vi "T1 new.vi"() -> ()   [LabVIEW 2012]
uses:
  <vilib>/DAQmx/read.llb/DAQmx Read (Counter U32 1Chan 1Samp).vi
  <vilib>/Analysis/1siggen.llb/Ramp Pattern by Samples.vi
  <vilib>/Utility/file.llb/Write To Spreadsheet File (DBL).vi
  <vilib>/Utility/file.llb/Write To Spreadsheet File (I64).vi
  <vilib>/DAQmx/create/channels.llb/DAQmx Create Channel (CI-Count Edges).vi
  <vilib>/DAQmx/configure/timing.llb/DAQmx Timing (Sample Clock).vi
  <vilib>/DAQmx/create/channels.llb/DAQmx Create Channel (CO-Pulse Generation-Ticks).vi
  <vilib>/DAQmx/configure/timing.llb/DAQmx Timing (Implicit).vi
  <vilib>/DAQmx/miscellaneous.llb/DAQmx Fill In Error Info.vi
  <resource>/objmgr/daqmx.rc
  <vilib>/Analysis/NI_AALBase.lvlib
panel:
  in  "N Cycles":i32
  in  "Sig/Ref Pause":dbl
  in  "file path (dialog if empty)":path
  in  "Z":dbl=0.001
  in  "Y":dbl=0.001
  in  "X":dbl=0.001
  out "Z Position":dbl=77.35
  out "Y Position":dbl=8.403706365395546
  out "X Position":dbl=39.29989668925261
  out "Cross Section Y":dbl[](graph)=[21.0, 21.0, 22.0, 23.0, 28.0, 18.0, 27.0, 23.0, 21.0, 23.0, 27.0, 24.0, 27.0, 48.0, 72.0, 155.0, 223.0, 269.0, 346.0, 310.0, 298.0, 201.0, 115.0, 77.0, 45.0, 31.0, 30.0, 22.0, 20.0, 22.0, 23.0, 32.0, 17.0, 24.0, 22.0, 22.0, 31.0, 30.0, 37.0]
  out "Cross Section X":dbl[](graph)=[40.0, 23.0, 29.0, 30.0, 20.0, 26.0, 17.0, 31.0, 49.0, 64.0, 98.0, 144.0, 182.0, 231.0, 269.0, 259.0, 260.0, 248.0, 193.0, 187.0, 133.0, 113.0, 84.0, 52.0, 39.0, 24.0, 24.0, 33.0, 19.0, 20.0, 16.0, 21.0, 26.0, 30.0, 25.0, 26.0, 20.0, 24.0, 24.0]
  out "Gave up?":bool
  in  "RS232 settings":cluster{"Portnumber":i32, "Baudrate":u16}={"Portnumber"=6, "Baudrate"=5} {"Portnumber" items=["COM1", "COM2", "COM3", "COM4", "COM5", "COM6", "COM7", "COM8", "COM9", "COM10", "COM11", "COM12", "COM13", "COM14", "COM15", "COM16", "COM17", "COM18", "COM19", "COM20", "COM21", "COM22", "COM23", "COM24", "COM25", "COM26", "COM27", "COM28", "COM29", "COM30"]; "Baudrate" items=["9600", "14400", "19200", "38400", "57600", "115200"]}
  in  "Y Parameters":T1={"Number of Y Steps"=200, "Max Y (V)"=2.0, "Min Y (V)"=-2.0}
  in  "X Parameters":T2={"Number of X Steps"=200, "Max X (V)"=2.0, "Min X (V)"=-2.0}
  in  "Path to spinapi.dll":path=path "C:/SpinCore/SpinAPI/dll/spinapi64.dll"
  in  "Pi Pulse?":bool
  in  "T1 AOM Rest":dbl=1e-06
  in  "Light Ratio":dbl=2.5e-06
  in  "T1 APD width":dbl=5e-07
  in  "T1 Signal Delay":dbl=6e-07
  in  "type 2":u16(ring)=1 items=["Linear", "Logarithmic"]
  in  "Tau No. Steps":i32=20
  in  "Tau Min":dbl=2e-08
  in  "Tau Max":dbl=0.001
  in  "Rabi Freq":dbl=7000000.0
  out "signal":u32
  out "ref":u32
  in  "samples per channel":i32=1000
  in  "N loops":i32=-1
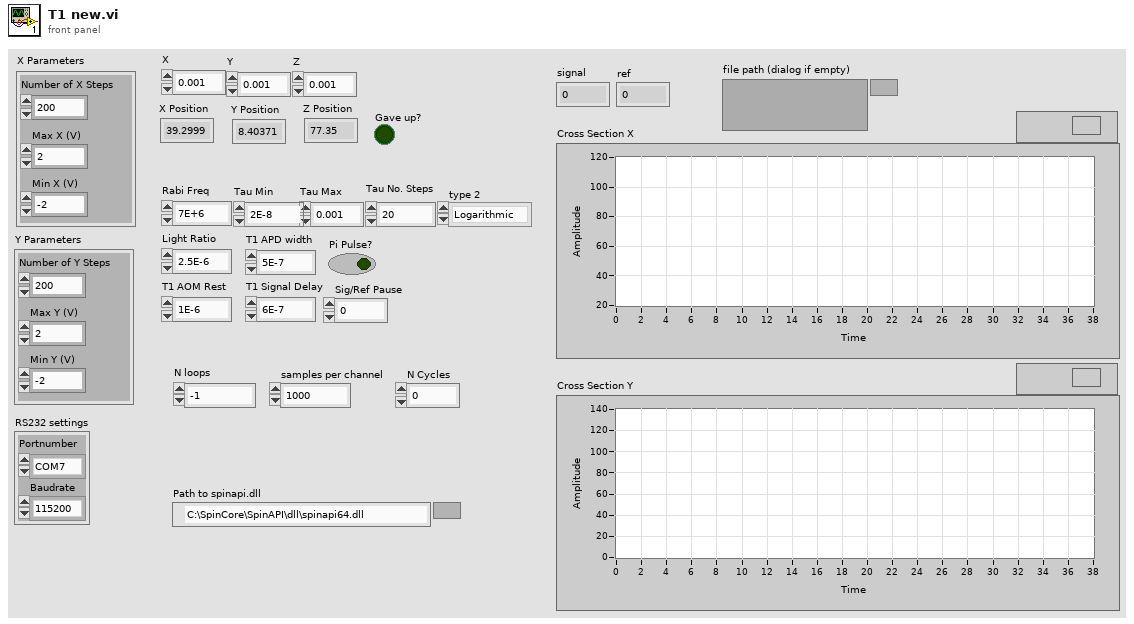
[diagram p1: front panel]
types:
  T1 = cluster{"Number of Y Steps":i32, "Max Y (V)":dbl, "Min Y (V)":dbl}
  T2 = cluster{"Number of X Steps":i32, "Max X (V)":dbl, "Min X (V)":dbl}
  T3 = enum16{"Pulse Program", "Frequency Registers", "TX Phase Registers", "RX Phase Registers"}
  T4 = cluster{"Instruct Data":i32, "Op Code":i32, "Flags":bool[], "Comments":string, "Time (s)":dbl}[]
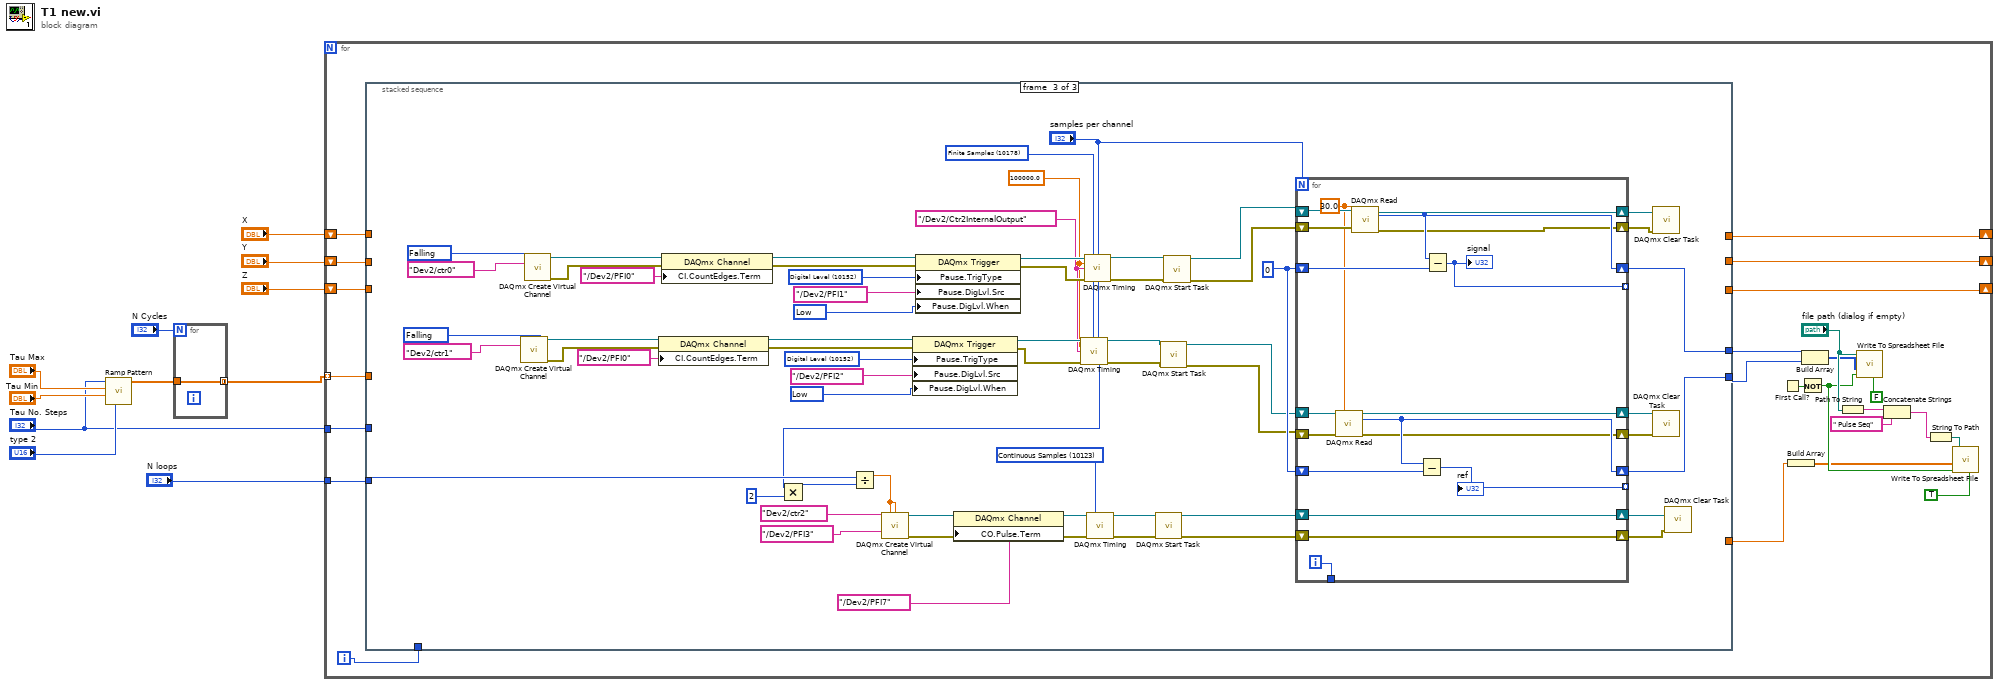
[diagram p0: block diagram]
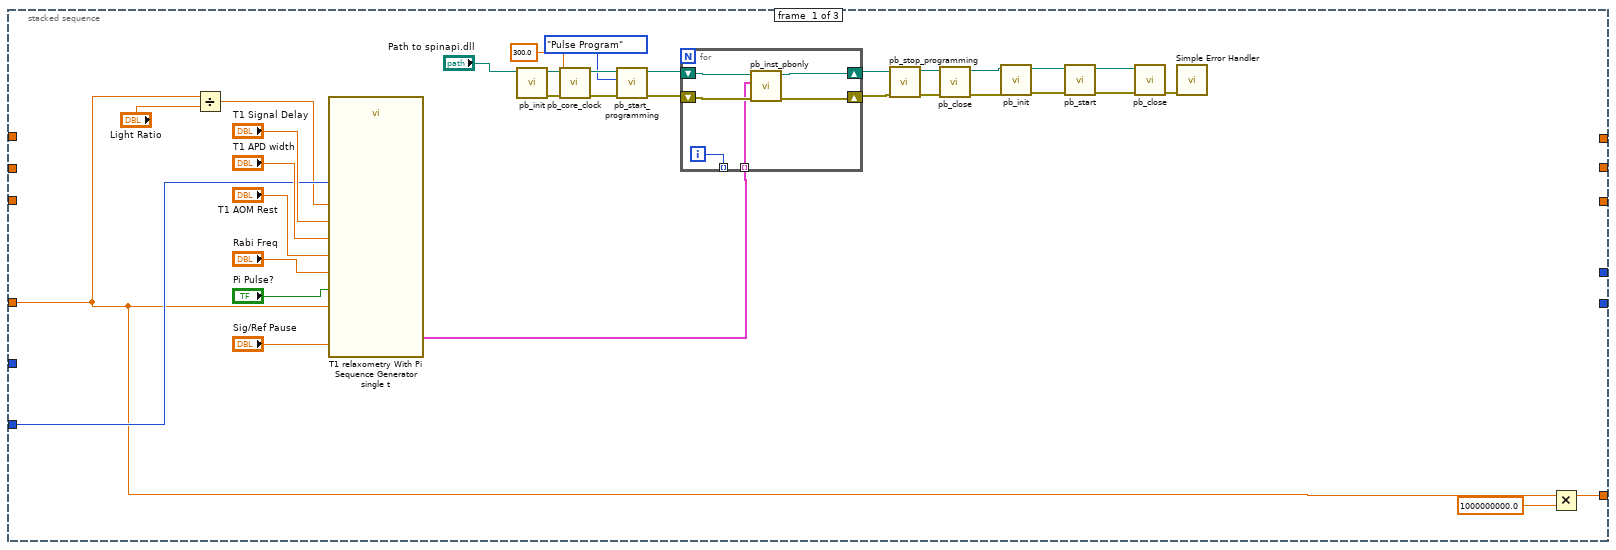
[diagram p2: hidden frame]
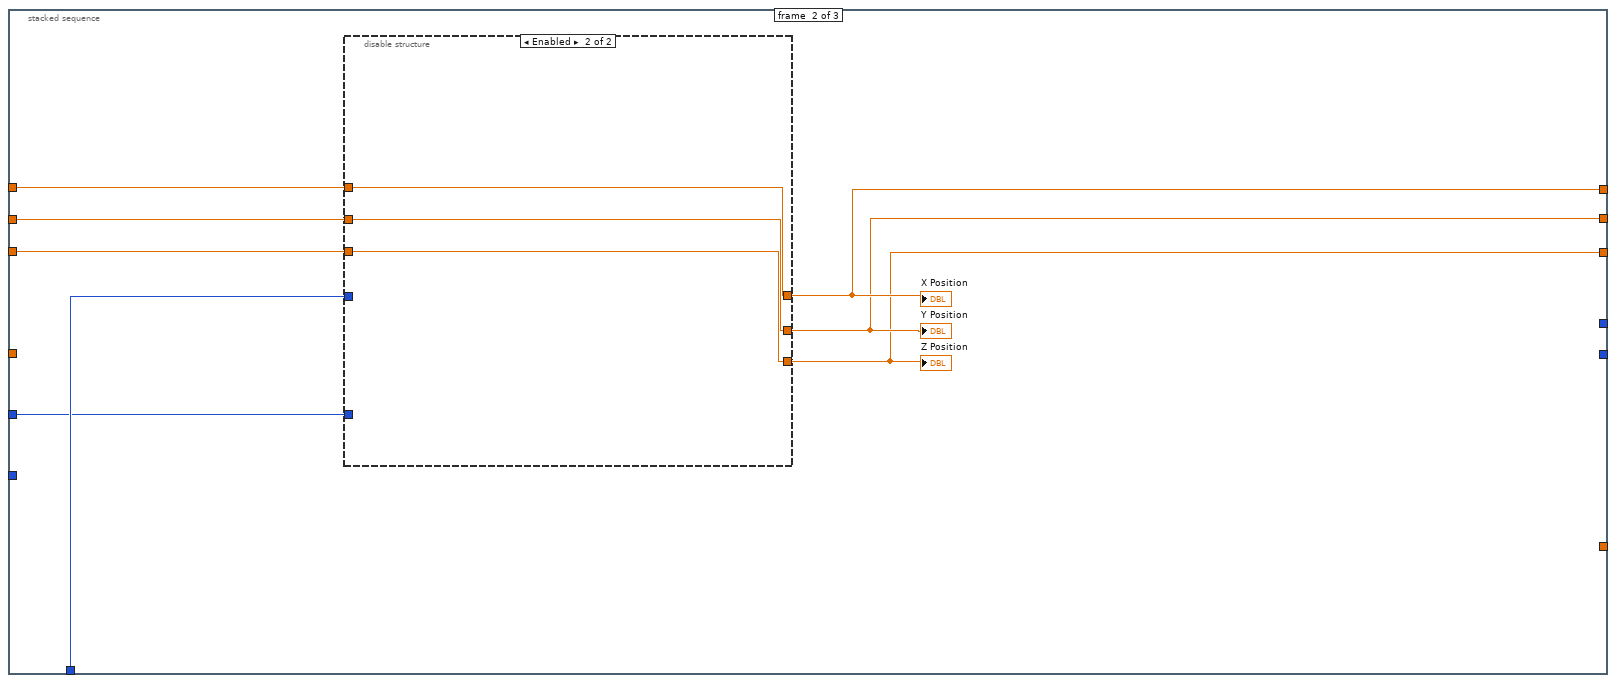
[diagram p3: hidden frame]
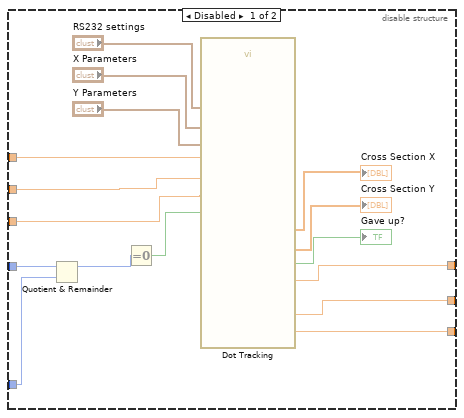
[diagram p4: hidden frame]
diagram:
  n1 = call-poly <vilib>:"Ramp Pattern.vi"("type"="type 2", "start"="Tau Min", "end"="Tau Max", "samples"="Tau No. Steps") -> ("Ramp Pattern"=w4:dbl[])  [unwired: 6 in, 1 out]
  n2 = for {
    N: "N Cycles" -> [_]
    tunnel: w4 -> [w12]
    tunnel: [w12] -> w3 mode=concatenating
  }
  n3 = for {
    tunnel: w3 -> [w36] mode=indexing
    tunnel: "N loops" -> [w35]
    shift-right: [w31] -> _
    shift-left: "X" -> [w34]
    shift-right: [w30] -> _
    shift-left: "Y" -> [w33]
    shift-right: [w29] -> _
    shift-left: "Z" -> [w32]
    tunnel: "Tau No. Steps" -> [w27]
    i -> [w28]
    n4 = stacked-sequence {
      tunnel: w36 -> [w39 _ _]
      tunnel: w35 -> [w64 _ w108]
      tunnel: w34 -> [_ w83 _]
      tunnel: w33 -> [_ w82 _]
      tunnel: w32 -> [_ w81 _]
      tunnel: [_ w80 _] -> w31
      tunnel: [_ w79 _] -> w30
      tunnel: [_ w78 _] -> w29
      tunnel: [_ _ w107] -> w19
      tunnel: [_ _ w106] -> w18
      tunnel: [w38 _ _] -> w14
      tunnel: w28 -> [_ w77 _]
      tunnel: w27 -> [_ w76 _]
      frame #0 {
        n5 = Divide(x=w39, y="Light Ratio") -> (x/y=w41:dbl)
        n6 = call "T1 relaxometry With Pi Sequence Generator single t.vi"("N Loop"=w64, "AOM Pulse length"=w41, "AOM Rest time"="T1 AOM Rest", "Signal Delay"="T1 Signal Delay", "APD signal width"="T1 APD width", "Tau"=w39, "Rabi Freq"="Rabi Freq", "Pi Pulse?"="Pi Pulse?", "Sig/Ref Pause"="Sig/Ref Pause") -> ("Array"=w50:T4)  [unwired: 10 in]
        n7 = call "pb_init.vi"("path in"="Path to spinapi.dll") -> ("error out"=w56:errorcluster, "path out"=w54:path)  [unwired: 3 in, 6 out]
        n8 = call "pb_core_clock.vi"("error in (no error)"=w56, "clock_freq (MHz)"=300.0, "path in"=w54) -> ("error out"=w57:errorcluster, "path out"=w55:path)  [unwired: 7 in]
        n9 = call "pb_start_programming.vi"("error in (no error)"=w57, "Device"=T3."Pulse Program", "path in"=w55) -> ("error out"=w60:errorcluster, "path out"=w59:path)  [unwired: 1 in, 6 out]
        n10 = for {
          shift-right: [w73] -> w61
          shift-left: w59 -> [w75]
          shift-right: [w72] -> w62
          shift-left: w60 -> [w74]
          tunnel: [w71] -> _ mode=indexing
          tunnel: w50 -> [w70] mode=indexing
          i -> [w71]
          n11 = call "pb_inst_pbonly.vi"("error in (no error)"=w74, "PB Instruction"=w70, "path in"=w75) -> ("error out"=w72:errorcluster, "path out"=w73:path)  [unwired: 2 in, 5 out]
        }
        n12 = call "pb_stop_programming.vi"("error in (no error)"=w62, "path in"=w61) -> ("error out"=w53:errorcluster, "path out"=w52:path)  [unwired: 1 in, 7 out]
        n13 = call "pb_close.vi"("error in (no error)"=w53, "path in"=w52) -> ("error out"=w48:errorcluster, "path out"=w45:path)  [unwired: 8 out]
        n14 = call "pb_init.vi"("error in (no error)"=w48, "path in"=w45) -> ("error out"=w47:errorcluster, "path out"=w44:path)  [unwired: 1 in, 7 out]
        n15 = call "pb_start.vi"("error in (no error)"=w47, "path in"=w44) -> ("error out"=w46:errorcluster, "path out"=w43:path)  [unwired: 1 in, 7 out]
        n16 = call "pb_close.vi"("error in (no error)"=w46, "path in"=w43) -> ("error out"=w49:errorcluster)  [unwired: 9 out]
        n17 = call <vilib>:"Simple Error Handler.vi"("error in (no error)"=w49) -> ()  [unwired: 1 in, 8 out]
        n18 = Multiply(x=w39, y=1000000000.0) -> (x*y=w38:dbl)
      }
      frame #1 {
        n19 = disable-structure shown="Enabled" {
          disable-tunnel: w83 -> [w93 w102]
          disable-tunnel: w82 -> [w92 w101]
          disable-tunnel: w81 -> [w91 w100]
          disable-tunnel: [w90 w102] -> w80
          disable-tunnel: [w89 w101] -> w79
          disable-tunnel: [w88 w100] -> w78
          disable-tunnel: w77 -> [w87 _]
          disable-tunnel: w76 -> [w86 _]
          frame Disabled {
            n20 = Quotient & Remainder(x=w87, y=w86) -> (x-y*floor(x/y)=w85:i32)  [unwired: 1 out]
            n21 = Equal To 0?(x=w85) -> (x = 0?=w84:bool)
            n22 = call "Dot Tracking.vi"("X"="X Parameters", "Y Parameters"="Y Parameters", "RS232 settings"="RS232 settings", "X Pos"=w93, "Y pos"=w92, "Z Pos"=w91, "Z-track?"=w84) -> ("X Position"=w90:dbl, "Y Position"=w89:dbl, "Z Position"=w88:dbl, "Cross Section X"=→"Cross Section X":dbl[], "Cross Section Y"=→"Cross Section Y":dbl[], "Gave up?"=→"Gave up?":bool)  [unwired: 2 in, 1 out]
          }
          frame Enabled {
          }
        }
        "X Position" <- w80
        "Y Position" <- w79
        "Z Position" <- w78
      }
      frame #2 {
        w121 = u32 0 ("data")
        w128 = 10123 items=["Finite Samples"=10178, "Continuous Samples"=10123, "Hardware Timed Single Point"=12522] ("sample mode")
        w145 = 10214 items=["High"=10192, "Low"=10214] ("Pause.DigLvl.When")
        w147 = 10152 items=["Analog Level"=10101, "Analog Window"=10103, "Digital Level"=10152, "Digital Pattern"=10398, "None"=10230] ("Pause.TrigType")
        w148 = 10171 items=["Rising"=10280, "Falling"=10171] ("edge")
        w109 = 10214 items=["High"=10192, "Low"=10214] ("Pause.DigLvl.When")
        w160 = 10152 items=["Analog Level"=10101, "Analog Window"=10103, "Digital Level"=10152, "Digital Pattern"=10398, "None"=10230] ("Pause.TrigType")
        w161 = 10171 items=["Rising"=10280, "Falling"=10171] ("edge")
        w125 = tag "/Dev2/Ctr2InternalOutput" ("source")
        w123 = 10178 items=["Finite Samples"=10178, "Continuous Samples"=10123, "Hardware Timed Single Point"=12522] ("sample mode")
        w124 = 100000.0 ("rate")
        n23 = call-poly <vilib>:"DAQmx Create Virtual Channel.vi"("edge"=w148, "counter"=tag "Dev2/ctr1") -> ("task out"=w143:refnum<k21>, "error out"=w140:errorcluster)  [unwired: 7 in, 5 out]
        n24 = call-poly <vilib>:"DAQmx Create Virtual Channel.vi"("edge"=w161, "counter"=tag "Dev2/ctr0") -> ("task out"=w157:refnum<k21>, "error out"=w154:errorcluster)  [unwired: 7 in, 5 out]
        n25 = property class="DAQmx Channel"(reference=w143, error in=w140, "CI.CountEdges.Term"=tag "/Dev2/PFI0") -> (reference out=w144:refnum<k21>, error out=w142:errorcluster)
        n26 = property class="DAQmx Channel"(reference=w157, error in=w154, "CI.CountEdges.Term"=tag "/Dev2/PFI0") -> (reference out=w158:refnum<k21>, error out=w156:errorcluster)
        n27 = Multiply(x="samples per channel", y=2) -> (x*y=w105:i32)
        n28 = Divide(x=w108, y=w105) -> (x/y=w133:dbl)
        n29 = call-poly <vilib>:"DAQmx Create Virtual Channel.vi"("high ticks"=w133, "low ticks"=w133, "counter"=tag "Dev2/ctr2", "source of ticks"=tag "/Dev2/PFI3" ("source")) -> ("task out"=w132:refnum<k21>, "error out"=w130:errorcluster)  [unwired: 10 in]
        n30 = property class="DAQmx Trigger"(reference=w144, error in=w142, "Pause.TrigType"=w147, "Pause.DigLvl.Src"=tag "/Dev2/PFI2", "Pause.DigLvl.When"=w145) -> (reference out=w139:refnum<k21>, error out=w138:errorcluster)
        n31 = property class="DAQmx Trigger"(reference=w158, error in=w156, "Pause.TrigType"=w160, "Pause.DigLvl.Src"=tag "/Dev2/PFI1", "Pause.DigLvl.When"=w109) -> (reference out=w153:refnum<k21>, error out=w152:errorcluster)
        n32 = property class="DAQmx Channel"(reference=w132, "CO.Pulse.Term"=tag "/Dev2/PFI7") -> (reference out=w127:refnum<k21>)  [unwired: 1 in, 1 out]
        n33 = call-poly <vilib>:"DAQmx Timing.vi"("task/channels in"=w139, "sample mode"=w123, "samples per channel"="samples per channel", "rate"=w124, "source"=w125, "error in"=w138) -> ("task out"=w137:refnum<k21>, "error out"=w136:errorcluster)  [unwired: 8 in]
        n34 = call-poly <vilib>:"DAQmx Timing.vi"("task/channels in"=w153, "sample mode"=w123, "samples per channel"="samples per channel", "rate"=w124, "source"=w125, "error in"=w152) -> ("task out"=w151:refnum<k21>, "error out"=w150:errorcluster)  [unwired: 8 in]
        n35 = call-poly <vilib>:"DAQmx Timing.vi"("task/channels in"=w127, "sample mode"=w128, "error in"=w130) -> ("task out"=w131:refnum<k21>, "error out"=w129:errorcluster)  [unwired: 11 in]
        n36 = call <vilib>:"DAQmx Start Task.vi"("task/channels in"=w131, "error in"=w129) -> ("task out"=w113:refnum<k21>, "error out"=w111:errorcluster)  [unwired: 12 in]
        n37 = call <vilib>:"DAQmx Start Task.vi"("task/channels in"=w137, "error in"=w136) -> ("task out"=w115:refnum<k21>, "error out"=w114:errorcluster)  [unwired: 12 out]
        n38 = call <vilib>:"DAQmx Start Task.vi"("task/channels in"=w151, "error in"=w150) -> ("task out"=w117:refnum<k21>, "error out"=w116:errorcluster)  [unwired: 12 out]
        n39 = for {
          N: "samples per channel" -> [_]
          shift-right: [w175] -> w120
          shift-left: w117 -> [w180]
          tunnel: [w177] -> _ mode=indexing
          shift-right: [w172] -> w107
          shift-left: w121 -> [w179]
          shift-right: [w173] -> w106
          shift-left: w121 -> [w178]
          shift-right: [w174] -> w122
          shift-left: w115 -> [w176]
          tunnel: [w171] -> _ mode=indexing
          shift-right: [w164] -> w119
          shift-left: w116 -> [w169]
          shift-right: [w170] -> w118
          shift-left: w114 -> [w168]
          tunnel: [w167] -> _
          shift-right: [w166] -> w112
          shift-left: w113 -> [w166]
          shift-right: [w165] -> w110
          shift-left: w111 -> [w165]
          i -> [w167]
          w163 = 30.0 ("timeout")
          n40 = call-poly <vilib>:"DAQmx Read.vi"("task/channels in"=w176, "timeout"=w163, "error in"=w168) -> ("task out"=w174:refnum<k21>, "data"=w173:u32, "error out"=w170:errorcluster)  [unwired: 10 in]
          n41 = call-poly <vilib>:"DAQmx Read.vi"("task/channels in"=w180, "timeout"=w163, "error in"=w169) -> ("task out"=w175:refnum<k21>, "data"=w172:u32, "error out"=w164:errorcluster)  [unwired: 10 in]
          n42 = Subtract(x=w173, y=w178) -> (x-y=w177:u32)
          "ref" <- w177
          n43 = Subtract(x=w172, y=w179) -> (x-y=w171:u32)
          "signal" <- w171
        }
        n44 = call <vilib>:"DAQmx Clear Task.vi"("task in"=w120, "error in"=w119) -> ()  [unwired: 13 in, 1 out]
        n45 = call <vilib>:"DAQmx Clear Task.vi"("task in"=w122, "error in"=w118) -> ()  [unwired: 13 in, 1 out]
        n46 = call <vilib>:"DAQmx Clear Task.vi"("task in"=w112, "error in"=w110) -> ()  [unwired: 13 in, 1 out]
      }
    }
    n47 = First Call?() -> (First Call?: T/F=w17:bool)
    n48 = Build Array(w14) -> (w13:dbl[])
    n49 = Not(x=w17) -> (.not. x?=w16:bool)
    n50 = Build Array(w19, w18) -> (w15:u32[])
    n51 = Path To String(path="file path (dialog if empty)") -> (string=w23:string)
    n52 = call-poly <vilib>:"Write To Spreadsheet File.vi"("transpose? (no:F)"=FALSE, "append to file? (new file:F)"=w16, "1D data"=w15, "file path (dialog if empty)"="file path (dialog if empty)") -> ()  [unwired: 4 in, 1 out]
    n53 = Concatenate Strings(w23, " Pulse Seq" ("string")) -> (w26:string)
    n54 = String To Path(string=w26) -> (path=w25:path)
    n55 = call-poly <vilib>:"Write To Spreadsheet File.vi"("transpose? (no:F)"=TRUE, "append to file? (new file:F)"=w16, "1D data"=w13, "file path (dialog if empty)"=w25) -> ()  [unwired: 4 in, 1 out]
  }
